vi "init butter.vi"(10 "butter":i32) -> (2 "init buffer":u16[](array[numeric]))   [LabVIEW 2009]
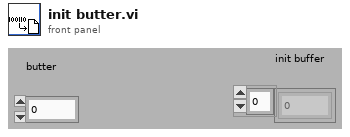
[diagram p1: front panel]
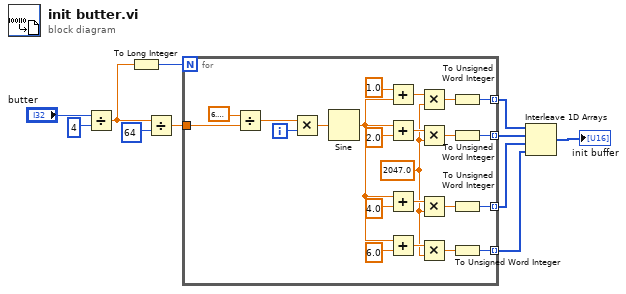
[diagram p0: block diagram]
diagram:
  n1 = Divide(x="butter", y=4) -> (x/y=w8:dbl)
  n2 = To Long Integer(number=w8) -> (32bit integer=w7:i32)
  n3 = Divide(x=w8, y=64) -> (x/y=w9:dbl)
  n4 = for {
    N: w7 -> [_]
    tunnel: [w30] -> w5 mode=indexing
    tunnel: w9 -> [w29]
    tunnel: [w14] -> w4 mode=indexing
    tunnel: [w13] -> w3 mode=indexing
    tunnel: [w12] -> w2 mode=indexing
    i -> [w33]
    w18 = 2047.0 ("y")
    n5 = Divide(x=6.283185307179586, y=w29) -> (x/y=w34:dbl)
    n6 = Multiply(x=w34, y=w33) -> (x*y=w32:dbl)
    n7 = Sine(x=w32) -> (sin(x)=w23:dbl)
    n8 = Add(x=1.0, y=w23) -> (x+y=w27:dbl)
    n9 = Add(x=w23, y=2.0) -> (x+y=w21:dbl)
    n10 = Add(x=w23, y=4.0) -> (x+y=w20:dbl)
    n11 = Add(x=w23, y=6.0) -> (x+y=w19:dbl)
    n12 = Multiply(x=w27, y=w18) -> (x*y=w26:dbl)
    n13 = Multiply(x=w21, y=w18) -> (x*y=w16:dbl)
    n14 = Multiply(x=w20, y=w18) -> (x*y=w15:dbl)
    n15 = Multiply(x=w19, y=w18) -> (x*y=w17:dbl)
    n16 = To Unsigned Word Integer(number=w26) -> (unsigned 16bit integer=w30:u16)
    n17 = To Unsigned Word Integer(number=w16) -> (unsigned 16bit integer=w14:u16)
    n18 = To Unsigned Word Integer(number=w15) -> (unsigned 16bit integer=w13:u16)
    n19 = To Unsigned Word Integer(number=w17) -> (unsigned 16bit integer=w12:u16)
  }
  n20 = Interleave 1D Arrays(w5, w4, w3, w2) -> (→"init buffer":u16[])
